vi "citTemplate.clearQueue.vi"(2 "instance (0)":i32, 7 "event in":variant, 11 "error in (no error)":errorcluster) -> (6 "Actions remaining":u32[](array[numeric]), 15 "error out":errorcluster)   [LabVIEW 2019, in "Tools.lvlib"]
uses:
  Tools.lvlib
  citTemplate.eventQueue.ctl
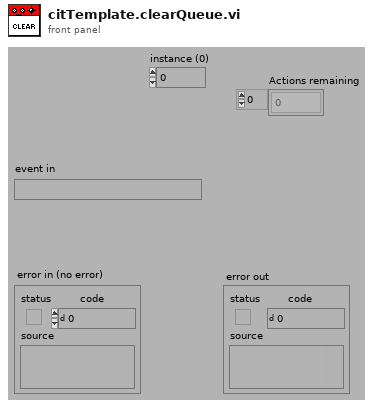
[diagram p1: front panel]
types:
  T1 = typedef "Tools.lvlib/citTemplate.eventQueue.ctl" = enum16{"create queue", "get queue handle(s)", "destroy queue"}
  T2 = typedef "ackNotifier.ctl" = refnum<notifier>
  T3 = cluster{"event index":u32, "(flatten) data in":string, "ack notifier":T2}[]
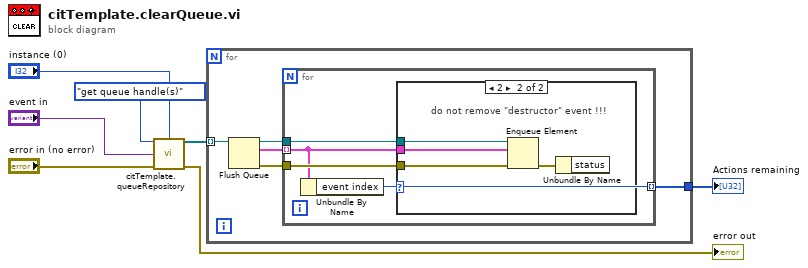
[diagram p0: block diagram]
diagram:
  n1 = call "citTemplate.queueRepository.vi"("mode (get queue handle)"=citTemplate.eventQueue."get queue handle(s)" ("mode (write event)"), "instance (0)"="instance (0)", "event in"="event in", "error in (no error)"="error in (no error)") -> ("queueHandle(s) out"=w4:refnum<queue>[], "error out"=→"error out":errorcluster)  [unwired: 2 in, 8 out]
  n2 = for {
    tunnel: w4 -> [w12] mode=indexing
    tunnel: [w8] -> w1
    n3 = Flush Queue(queue=w12) -> (queue out=w10:refnum<queue>, remaining elements=w11:T3, error out=w9:errorcluster)  [unwired: 1 in]
    n4 = for {
      tunnel: w11 -> [w14] mode=indexing
      tunnel: w10 -> [w16]
      tunnel: w9 -> [w15]
      tunnel: [w13] -> w8 mode=indexing
      n5 = Unbundle By Name(w14) -> ("event index"=w13:u32)
      n6 = case shown="2" w13 {
        tunnel: w16 -> [_ w20]
        tunnel: w15 -> [_ w19]
        tunnel: w14 -> [_ w17]
        frame Default {
        }
        frame 2 {
          # "do not remove \"destructor\" event !!!"
          n7 = Enqueue Element(queue=w20, element=w17, error in (no error)=w19) -> (error out=w18:errorcluster)  [unwired: 3 out]
          n8 = Unbundle By Name(w18) -> ()  [unwired: 1 out]
        }
      }
    }
  }
  "Actions remaining" <- w1
